vi "Get Interface Configuration.vi"(8 "error in (no error)":errorcluster, 10 "Configuration Parameter (RS-232 Enable/Disable)":i32(ring) items=["RS-232 Enable/Disable", "RS-232 Baud Rate", "GPIB Enable/Disable", "GPIB Address", "LAN TCP/IP Enable/Disable", "DHCP Enable/Disable", "Auto-Ip Enable/Disable", "Static Ip Enable/Disable", "Bare Socket Enable/Disable", "Telnet Enable/Disable", "VXI-11 Net Instrument Enable/Disable", "Static IP Address", "Subnet Address/Network Mask", "Default Gateway"], 11 "VISA resource name":refnum<visa-resource-name>) -> (0 "error out":errorcluster, 2 "Value":string, 3 "VISA resource name out":refnum<visa-resource-name>, 4 "Device Errors":cluster{"code":i32, "Text":string}[](array[cluster]))   [LabVIEW 2014, in "Stanford Research DG645 - Driver.lvlib"]
doc: "Interface Command: IFCF? i\nInstrument Error Check\n\nQuery the interface configuration parameter. The parameter i may be one of the following:\n\ni Configuration Parameter\n0 RS-232 Enable/Disable\n1 RS-232 Baud rate\n2 GPIB Enable/Disable\n3 GPIB Address\n4 LAN TCP/IP Enable/Disable\n5 DHCP Enable/Disable\n6 Auto-Ip Enable/Disable\n7 Static Ip Enable/Disable\n8 Bare Socket Enable/Disable\n9 Telnet Enable/Disable\n10 VXI-11 Net Instrument Enable/Disable\n11 Static IP Address\n12 Subnet Address/Network Mask\n13 Default Gateway\n\n1 means enabled, 0 disabled."
uses:
  Stanford Research DG645 - Driver.lvlib
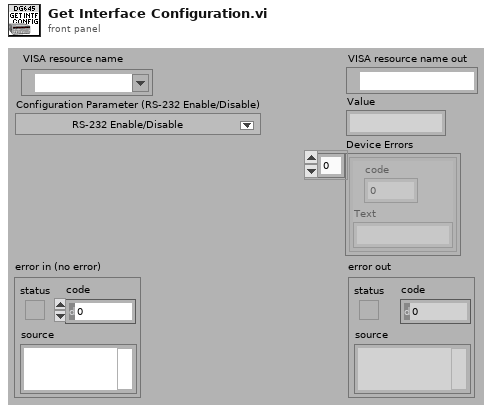
[diagram p1: front panel]
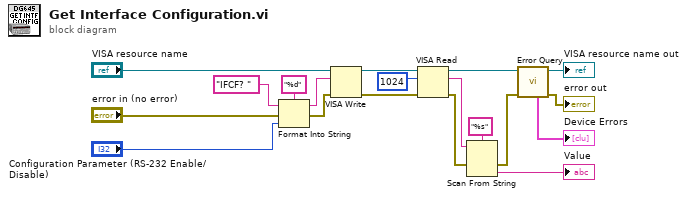
[diagram p0: block diagram]
diagram:
  n1 = Format Into String(format string="%d", initial string="IFCF? " ("command"), error in="error in (no error)", "Configuration Parameter (RS-232 Enable/Disable)") -> (resulting string=w2:string, error out=w3:errorcluster)
  n2 = VISA Write(VISA resource name="VISA resource name", write buffer=w2, error in (no error)=w3) -> (VISA resource name out=w11:refnum<visa-resource-name>, error out=w9:errorcluster)  [unwired: 1 out]
  n3 = VISA Read(VISA resource name=w11, byte count=u32 1024, error in (no error)=w9) -> (VISA resource name out=w10:refnum<visa-resource-name>, read buffer=w13:string, error out=w12:errorcluster)  [unwired: 1 out]
  n4 = Scan From String(format string="%s", input string=w13, error in=w12) -> (error out=w8:errorcluster, output 1=→"Value":string)  [unwired: 2 in, 2 out]
  n5 = call "Error Query.vi"("error in (no error)"=w8, "VISA resource name"=w10) -> ("error out"=→"error out":errorcluster, "VISA resource name out"=→"VISA resource name out":refnum<visa-resource-name>, "Device Errors"=→"Device Errors":cluster{"code":i32, "Text":string}[])  [unwired: 7 in]
